vi "Pack1 Cluster and Padding Cluster.vi"() -> ()   [LabVIEW 2012]
uses:
  demo dll.dll
panel:
  out "CStructNoPack":T1
  out "Pack1Cluster":cluster{"U8":u8, "I32":i32, "DBL":dbl}
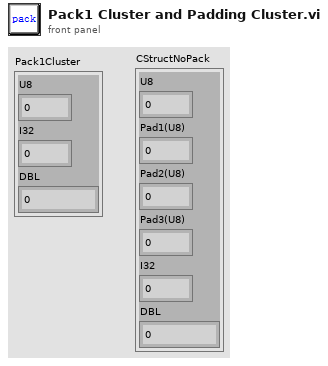
[diagram p1: front panel]
types:
  T1 = cluster{"U8":u8, "Pad1(U8)":u8, "Pad2(U8)":u8, "Pad3(U8) ":u8, "I32":i32, "DBL":dbl}
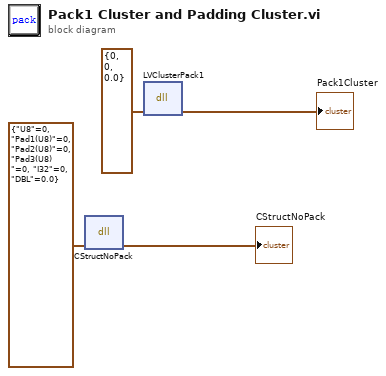
[diagram p0: block diagram]
diagram:
  n1 = dll-call lib="PTH1+abs EBOOK\t功能块DLLdemo dll.dll" fn="CStructNoPack"("CStructNoPack"=T1 {"U8"=0, "Pad1(U8)"=0, "Pad2(U8)"=0, "Pad3(U8) "=0, "I32"=0, "DBL"=0.0}) -> ("CStructNoPack"=→"CStructNoPack":T1)  [unwired: 4 in, 2 out]
  n2 = dll-call lib="PTH1+abs EBOOK\t功能块DLLdemo dll.dll" fn="LVClusterPack1"("Pack1Cluster"=cluster{"U8":u8, "I32":i32, "DBL":dbl} {"U8"=0, "I32"=0, "DBL"=0.0}) -> ("Pack1Cluster"=→"Pack1Cluster":cluster{"U8":u8, "I32":i32, "DBL":dbl})  [unwired: 4 in, 2 out]
